vi "load.vi"(8 "error in (no error)":errorcluster, 10 "index":i32, 11 "AnalysisRAPS in":refnum<class "AnalysisRAPS.lvclass">) -> (0 "error out":errorcluster, 3 "AnalysisRAPS out":refnum<class "AnalysisRAPS.lvclass">)   [LabVIEW 2010, in "AnalysisRAPS.lvclass"]
uses:
  AnalysisRAPS.lvclass
  AnalysisRAPS.lvclass/AnalysisRAPS.ctl
  common/classes/ImageCollection/ImageCollection/ImageCollection.lvclass
  common/classes/Image/Image/Image.lvclass
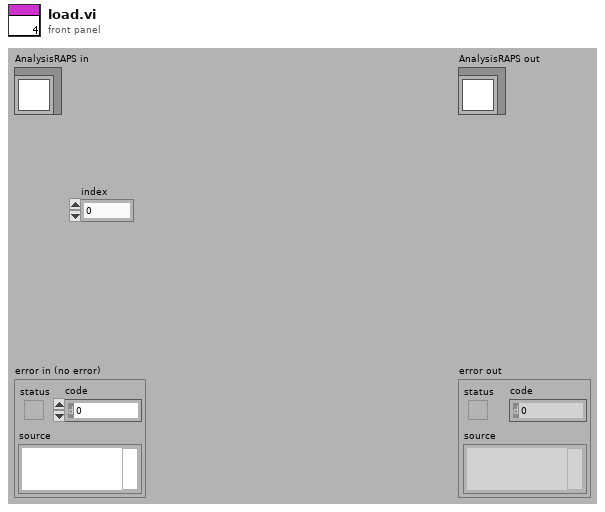
[diagram p1: front panel]
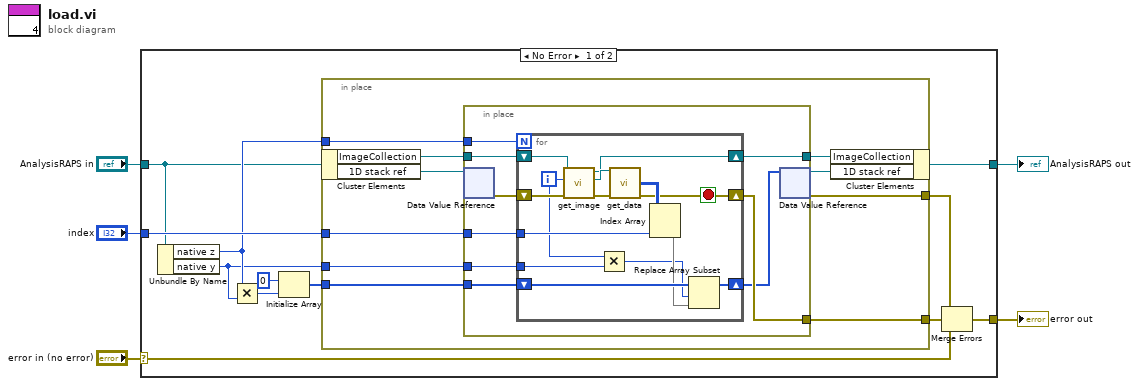
[diagram p0: block diagram]
diagram:
  n1 = case shown="No Error" "error in (no error)" {
    selector: "error in (no error)" -> [w6 w52]
    tunnel: [w15 w52] -> w4
    tunnel: [w7 w51] -> w2
    tunnel: "AnalysisRAPS in" -> [w8 w51]
    tunnel: "index" -> [w14 _]
    frame No Error {
      n2 = Unbundle By Name(w8) -> ("native z"=w13:i32, "native y"=w9:i32)
      n3 = Multiply(x=w13, y=w9) -> (x*y=w12:i32)
      n4 = Initialize Array(u16 0, w12) -> (w10:u16[])
      n5 = in-place {
        in-place-border: [w27] -> w17
        in-place-border: [w26] -> w16
        in-place-border: w14 -> [w25]
        in-place-border: w13 -> [w24]
        in-place-border: w10 -> [w23]
        in-place-border: w9 -> [w22]
        n6 = in-place-cluster #1(w8) -> ("ImageCollection"=w21:refnum<class "ImageCollection.lvclass">, "1D stack ref"=w19:refnum<data-value>)
        n7 = in-place {
          in-place-border: [w35] -> w26
          in-place-border: w21 -> [w36]
          in-place-border: w24 -> [w32]
          in-place-border: w25 -> [w33]
          in-place-border: w23 -> [w31]
          in-place-border: w22 -> [w30]
          in-place-border: [w29] -> w20
          n8 = in-place-dvr #2(w19) -> (w34:errorcluster)  [unwired: 1 out]
          n9 = for {
            N: w32 -> [_]
            shift-right: [w38] -> w35
            shift-left: w34 -> [w47]
            shift-right: [w37] -> w29
            shift-left: w36 -> [w50]
            tunnel: w33 -> [w45]
            shift-right: [w43] -> w28
            shift-left: w31 -> [w44]
            tunnel: w30 -> [w40]
            i -> [w41]
            stop <- w38 stop-if-true
            n10 = call-dynamic "get_image.vi"("error in (no error)"=w47, "index"=w41, "ImageCollection in"=w50) -> ("error out"=w48:errorcluster, "Image.lvclass"=w49:refnum<class "Image.lvclass">, "ImageCollection out"=w37:refnum<class "ImageCollection.lvclass">)  [unwired: 6 in]
            n11 = Multiply(x=w41, y=w40) -> (x*y=w39:i32)
            n12 = call-dynamic "get_data.vi"("Image in"=w49, "error in (no error)"=w48) -> ("Image Pixels (U16)"=w46:u16[][], "error out"=w38:errorcluster)  [unwired: 5 in, 7 out]
            n13 = Index Array(array=w46, index (col)=w45) -> (element=w42:u16[])  [unwired: 1 in]
            n14 = Replace Array Subset(array=w44, new element=w42, index=w39) -> (w43:u16[])
          }
          n15 = in-place-dvr #2(w28) -> (w18:refnum<data-value>, w27:errorcluster)
        }
        n16 = in-place-cluster #1("ImageCollection"=w20, "1D stack ref"=w18) -> (w7:refnum<class "AnalysisRAPS.lvclass">)
      }
      n17 = Merge Errors(w17, w16, w6) -> (w15:errorcluster)
    }
    frame Error {
    }
  }
  "error out" <- w4
  "AnalysisRAPS out" <- w2
